vi "CollideWithSquare.vi"(8 "error in (no error)":errorcluster, 10 "Square":T2, 11 "GameObject in":refnum<class "GameObject.lvclass">) -> (0 "error out":errorcluster, 1 "direction_y":T1, 2 "direction_x":T1, 3 "GameObject out":refnum<class "GameObject.lvclass">)   [LabVIEW 2019, in "RT_Game.lvlib" / "GameObject.lvclass"]
uses:
  GameObject.lvclass
  Square.ctl
  Game/Coordinate.ctl
  Direction.ctl
  GameObject.lvclass/GameObject.ctl
  RT_Game.lvlib
  Game/Game.lvclass
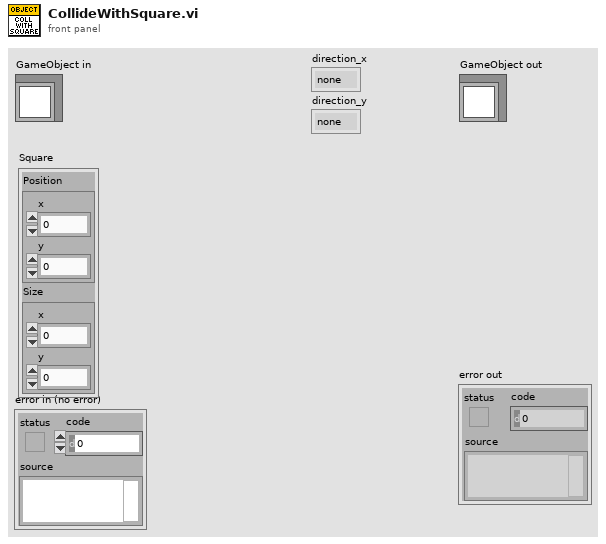
[diagram p1: front panel]
types:
  T1 = typedef "RT_Game.lvlib/Direction.ctl" = enum16{"none", "Both", "left", "right", "up", "down"}
  T2 = typedef "RT_Game.lvlib/Square.ctl" = cluster{"Position":T3, "Size":T3}
  T3 = typedef "RT_Game.lvlib/Game.lvclass/Coordinate.ctl" = cluster{"x":dbl, "y":dbl}
  T4 = typedef "RT_Game.lvlib/Velocity.ctl" = cluster{"x":dbl, "y":dbl}
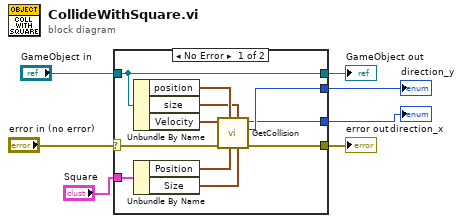
[diagram p0: block diagram]
diagram:
  n1 = case shown="No Error" "error in (no error)" {
    selector: "error in (no error)" -> [w18 w20]
    tunnel: [w16 w20] -> w6
    tunnel: [w15 w19] -> w4
    tunnel: "GameObject in" -> [w15 w19]
    tunnel: "Square" -> [w17 _]
    tunnel: [w9 _] -> w2
    tunnel: [w8 _] -> w1
    frame No Error {
      n2 = Unbundle By Name(w15) -> ("position"=w13:T3, "size"=w12:T3, "Velocity"=w14:T4)
      n3 = Unbundle By Name(w17) -> ("Position"=w11:T3, "Size"=w10:T3)
      n4 = call "GetCollision.vi"("TheirSize"=w10, "MySize"=w12, "TheirPosition"=w11, "MyPosition"=w13, "error in (no error)"=w18, "Velocity"=w14) -> ("error out"=w16:errorcluster, "direction_y"=w9:T1, "direction_x"=w8:T1)  [unwired: 3 in]
    }
    frame Error {
    }
  }
  "error out" <- w6
  "GameObject out" <- w4
  "direction_x" <- w1
  "direction_y" <- w2
